vi "GV DO gate.vi"() -> ()   [LabVIEW 2017]
panel:
  out "DO gate":bool
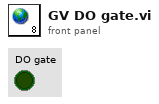
[diagram p1: front panel]
diagram:
